vi "Main.vi"(11 "Module Admin":refnum<class "Delacor_lib_QMH_Module Admin.lvclass">) -> ()   [LabVIEW 2023, in "RT Main.lvlib"]
doc: "This template is based off of the Queued Message Handler design pattern and the Queued Message Handler project template that ships with LabVIEW.\n\nThe main difference is that the queue is private to this module and communication between modules is performed via Broadcast and Request events.\n\nRequest events are wrapped in public API methods and are handled in the Event Handling Loop (EHL) of this VI. Any module can register for Broadcast events sent by this module. The EHL generates messages based on user interface actions.\n\nThe Message Handling Loop (MHL) processes messages generated by the EHL, or by other messages. The messages are string values, so new messages can be added easily to the Message Cases case structure in the MHL. Each message cluster can also provide an optional value for Message Data, which is a variant that can be converted to whatever message-specific data is required.\n_____\nBased on DQMH Dev Tools: Project Template 7.1.2.1547."
uses:
  RT Main.lvlib
  <vilib>/Delacor/Delacor QMH/Libraries/Module Admin_class/Delacor_lib_QMH_Module Admin.lvclass
  Module Data--cluster.ctl
  <vilib>/myRIO/Instrument Drivers/Onboard IO/AI/typedefs/AI Reference.ctl
  <vilib>/myRIO/Common/Instrument Driver Framework/Utilities/typedefs/myRIO Generic Hardware Reference.ctl
  <vilib>/myRIO/Common/Instrument Driver Framework/Utilities/typedefs/Hardware Version Enum.ctl
  <vilib>/myRIO/Common/Instrument Driver Framework/Utilities/typedefs/myRIO v1.0 Reference.ctl
  <vilib>/myRIO/Common/Instrument Driver Framework/Utilities/typedefs/Generic FPGA Reference.ctl
  <vilib>/myRIO/Common/Instrument Driver Framework/myRIO v1.0/AI/typedefs/AI Channels List.ctl
  <vilib>/myRIO/Common/Instrument Driver Framework/myRIO v1.0/AI/typedefs/AI Channels Enum.ctl
  <vilib>/myRIO/Common/Instrument Driver Framework/Utilities/typedefs/Analog Scaling Constants List.ctl
  <vilib>/myRIO/Common/Instrument Driver Framework/Utilities/typedefs/Analog Scaling Constants.ctl
  <vilib>/myRIO/Instrument Drivers/Onboard IO/DIO/typedefs/DIO Reference.ctl
  <vilib>/myRIO/Common/Instrument Driver Framework/myRIO v1.0/DIO/typedefs/DIO Channels List.ctl
  <vilib>/myRIO/Common/Instrument Driver Framework/myRIO v1.0/DIO/typedefs/DIO Channels Enum.ctl
  Modules Launched.ctl
  Hardware Monitoring.ctl
  Stop Argument--cluster.ctl
  <vilib>/Delacor/Delacor QMH/Libraries/Message Queue_class/Delacor_lib_QMH_Message Queue.lvclass/Delacor_lib_QMH_Message Queue.ctl
  <vilib>/Delacor/Delacor QMH/Libraries/Module Admin_class/Delacor_lib_QMH_Module Admin.lvclass/Delacor_lib_QMH_Module Admin.ctl
  Control Loop Cluster.ctl
  Data Cluster.ctl
  <vilib>/Delacor/Delacor QMH/Libraries/Message Queue_class/Delacor_lib_QMH_Enqueue Message (Single).vi
  <vilib>/Delacor/Delacor QMH/Libraries/Module Admin_class/Delacor_lib_QMH_Get External Launch.vi
  <vilib>/nisyscfg/Close (System).vi
  Control Loop.vi
  <vilib>/Delacor/Delacor QMH/Libraries/Message Queue_class/Delacor_lib_QMH_Message Queue.lvclass
  Analog Input/Analog Input.lvlib
  <vilib>/myRIO/Instrument Drivers/Onboard IO/AI/AI.lvlib
  <vilib>/nisyscfg/nisyscfg.lvlib
  <resource>/objmgr/nicriosae.rc
  <resource>/objmgr/nisysapi.rc
  Digital Inputs/Digital Inputs.lvlib
  <vilib>/myRIO/Instrument Drivers/Onboard IO/DIO/DIO.lvlib
  Modules/TDMS/TDMS.lvlib
  UDP RT/UDP RT.lvlib
panel:
  out "error out":errorcluster
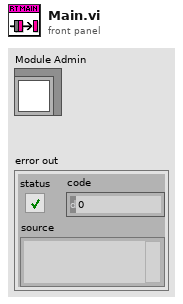
[diagram p1: front panel]
types:
  T1 = typedef "RT Main.lvlib/Request Events--cluster.ctl" = cluster{"Stop Module":refnum<user-event>, "Show Panel":refnum<user-event>, "Hide Panel":refnum<user-event>, "Get Module Execution Status":refnum<user-event>, "Show Diagram":refnum<user-event>, "Private.Launch Control Loop":refnum<user-event>, "Private.RT FIFO Ref":refnum<user-event>}
  T2 = typedef "Analog Input.lvlib/Broadcast Events--cluster.ctl" = cluster{"Module Did Init":refnum<user-event>, "Status Updated":refnum<user-event>, "Error Reported":refnum<user-event>, "Module Did Stop":refnum<user-event>, "Update Module Execution Status":refnum<user-event>, "AI Input Reference":refnum<user-event>}
  T3 = typedef "Digital Inputs.lvlib/Broadcast Events--cluster.ctl" = cluster{"Module Did Init":refnum<user-event>, "Status Updated":refnum<user-event>, "Error Reported":refnum<user-event>, "Module Did Stop":refnum<user-event>, "Update Module Execution Status":refnum<user-event>, "Send DI Reference":refnum<user-event>}
  T4 = typedef "TDMS.lvlib/Broadcast Events--cluster.ctl" = cluster{"Module Did Init":refnum<user-event>, "Status Updated":refnum<user-event>, "Error Reported":refnum<user-event>, "Module Did Stop":refnum<user-event>, "Update Module Execution Status":refnum<user-event>}
  T5 = typedef "UDP RT.lvlib/Broadcast Events--cluster.ctl" = cluster{"Module Did Init":refnum<user-event>, "Status Updated":refnum<user-event>, "Error Reported":refnum<user-event>, "Module Did Stop":refnum<user-event>, "Update Module Execution Status":refnum<user-event>, "Send UDP Info to TL":refnum<user-event>}
  T6 = typedef "RT Main.lvlib/Module Data--cluster.ctl" = cluster{"Status":string, "Current Directory":path, "AI Reference":T7, "DIO Reference":T16, "UDP Info":cluster{"IP Host":string, "Port RT":u16, "Port Host":u16, "connection ID":refnum<k16>}, "Modules Launched":T19, "RTFIFO HW":refnum<k33>}
  T7 = typedef "AI.lvlib/AI Reference.ctl" = cluster{"myRIO Reference":T8, "AI Channels List":T12, "AI Scaling Constants List":T14}
  T8 = typedef "myRIO Generic Hardware Reference.ctl" = cluster{"myRIO Model":T9, "myRIO Hardware Reference":T10}
  T9 = typedef "Hardware Version Enum.ctl" = enum16{"Unknown", "myRIO-1900", "myRIO-1950", "roboRIO", "NI ELVIS RIO CM", "ELVIS III"}
  T10 = typedef "myRIO v1.0 Reference.ctl" = cluster{"Generic FPGA Reference":T11, "Allow multiple opens":bool}
  T11 = typedef "Generic FPGA Reference.ctl" = refnum<k20>
  T12 = typedef "AI Channels List.ctl" = T13[]
  T13 = typedef "AI Channels Enum.ctl" = enum16{"Not Connected", "AudioIn/Left", "AudioIn/Right", "C/AI0", "C/AI1", "A/AI0", "A/AI1", "A/AI2", "A/AI3", "A/AI4", "A/AI5", "A/AI6", "A/AI7", "B/AI0", "B/AI1", "B/AI2", "B/AI3", "B/AI4", "B/AI5", "B/AI6", "B/AI7", "AI/AI0", "AI/AI1", "AI/AI2", "AI/AI3", "A/AI0 (DIFF)", "A/AI1 (DIFF)", "A/AI2 (DIFF)", "A/AI3 (DIFF)", "B/AI0 (DIFF)", "B/AI1 (DIFF)", "B/AI2 (DIFF)", "B/AI3 (DIFF)"}
  T14 = typedef "Analog Scaling Constants List.ctl" = T15[]
  T15 = typedef "Analog Scaling Constants.ctl" = cluster{"LSB Weight (Volts)":dbl, "Offset (Volts)":dbl, "Signed?":bool}
  T16 = typedef "DIO.lvlib/DIO Reference.ctl" = cluster{"myRIO Reference":T8, "DIO Channels List":T17}
  T17 = typedef "DIO Channels List.ctl" = T18[]
  T18 = typedef "DIO Channels Enum.ctl" = enum16{"Not Connected", "C/DIO0", "C/DIO1", "C/DIO2", "C/DIO3", "C/DIO4", "C/DIO5", "C/DIO6", "C/DIO7", "A/DIO0", "A/DIO1", "A/DIO2", "A/DIO3", "A/DIO4", "A/DIO5", "A/DIO6", "A/DIO7", "A/DIO8", "A/DIO9", "A/DIO10", "A/DIO11", "A/DIO12", "A/DIO13", "A/DIO14", "A/DIO15", "A/DIO16", "A/DIO17", "A/DIO18", "A/DIO19", "B/DIO0", "B/DIO1", "B/DIO2", "B/DIO3", "B/DIO4", "B/DIO5", "B/DIO6", "B/DIO7", "B/DIO8", "B/DIO9", "B/DIO10", "B/DIO11", "B/DIO12", "B/DIO13", "B/DIO14", "B/DIO15", "B/DIO16", "B/DIO17", "B/DIO18", "B/DIO19", "LED0", "LED1", "LED2", "LED3", "Button0", "DIO/DIO0", "DIO/DIO1", "DIO/DIO2", "DIO/DIO3", "DIO/DIO4", "DIO/DIO5", "DIO/DIO6", "DIO/DIO7", "DIO/DIO8", "DIO/DIO9", "SPI/CS0", "SPI/CS1", "SPI/CS2", "SPI/CS3", "LED RADIO (Green)", "LED RADIO (Red)", "LED COMM (Green)", "LED COMM (Red)", "LED MODE (Green)", "LED MODE (Red)"}
  T19 = typedef "RT Main.lvlib/Modules Launched.ctl" = cluster{"AI Input":bool, "DI Input":bool, "TDMS Module":bool, "UDP Module":bool}
  T20 = typedef "RT Main.lvlib/Hardware Monitoring.ctl" = cluster{"Memory RAM Free (%)":dbl, "Memory ROM Free (%)":dbl, "CPU 1 (%)":u32, "CPU 2 (%)":u32}
  T21 = enum32{"invalid lock state", "Not Locked", "Locked (No Password)", "Password-protected"}
  T22 = typedef "RT Main.lvlib/Stop Argument--cluster.ctl" = cluster{"Origin":string, "Exit via Stop Module Req?":bool, "Wait for Module to stop?":bool}
  T23 = cluster{"IP Host":string, "Port RT":u16, "Port Host":u16, "connection ID":refnum<k16>}
  T24 = typedef "RT Main.lvlib/Control Loop Cluster.ctl" = cluster{"AI Reference":T7, "DIO Reference":T16, "Data Cluster":T25, "TDMS Record?":bool, "Writing?":bool, "UDP Info":cluster{"IP Host":string, "Port RT":u16, "Port Host":u16, "connection ID":refnum<k16>}, "RT FIFO HW":refnum<k33>}
  T25 = typedef "RT Main.lvlib/Data Cluster.ctl" = cluster{"Analog Input":dbl[], "Digital Inputs":bool[], "U32":u32[]}
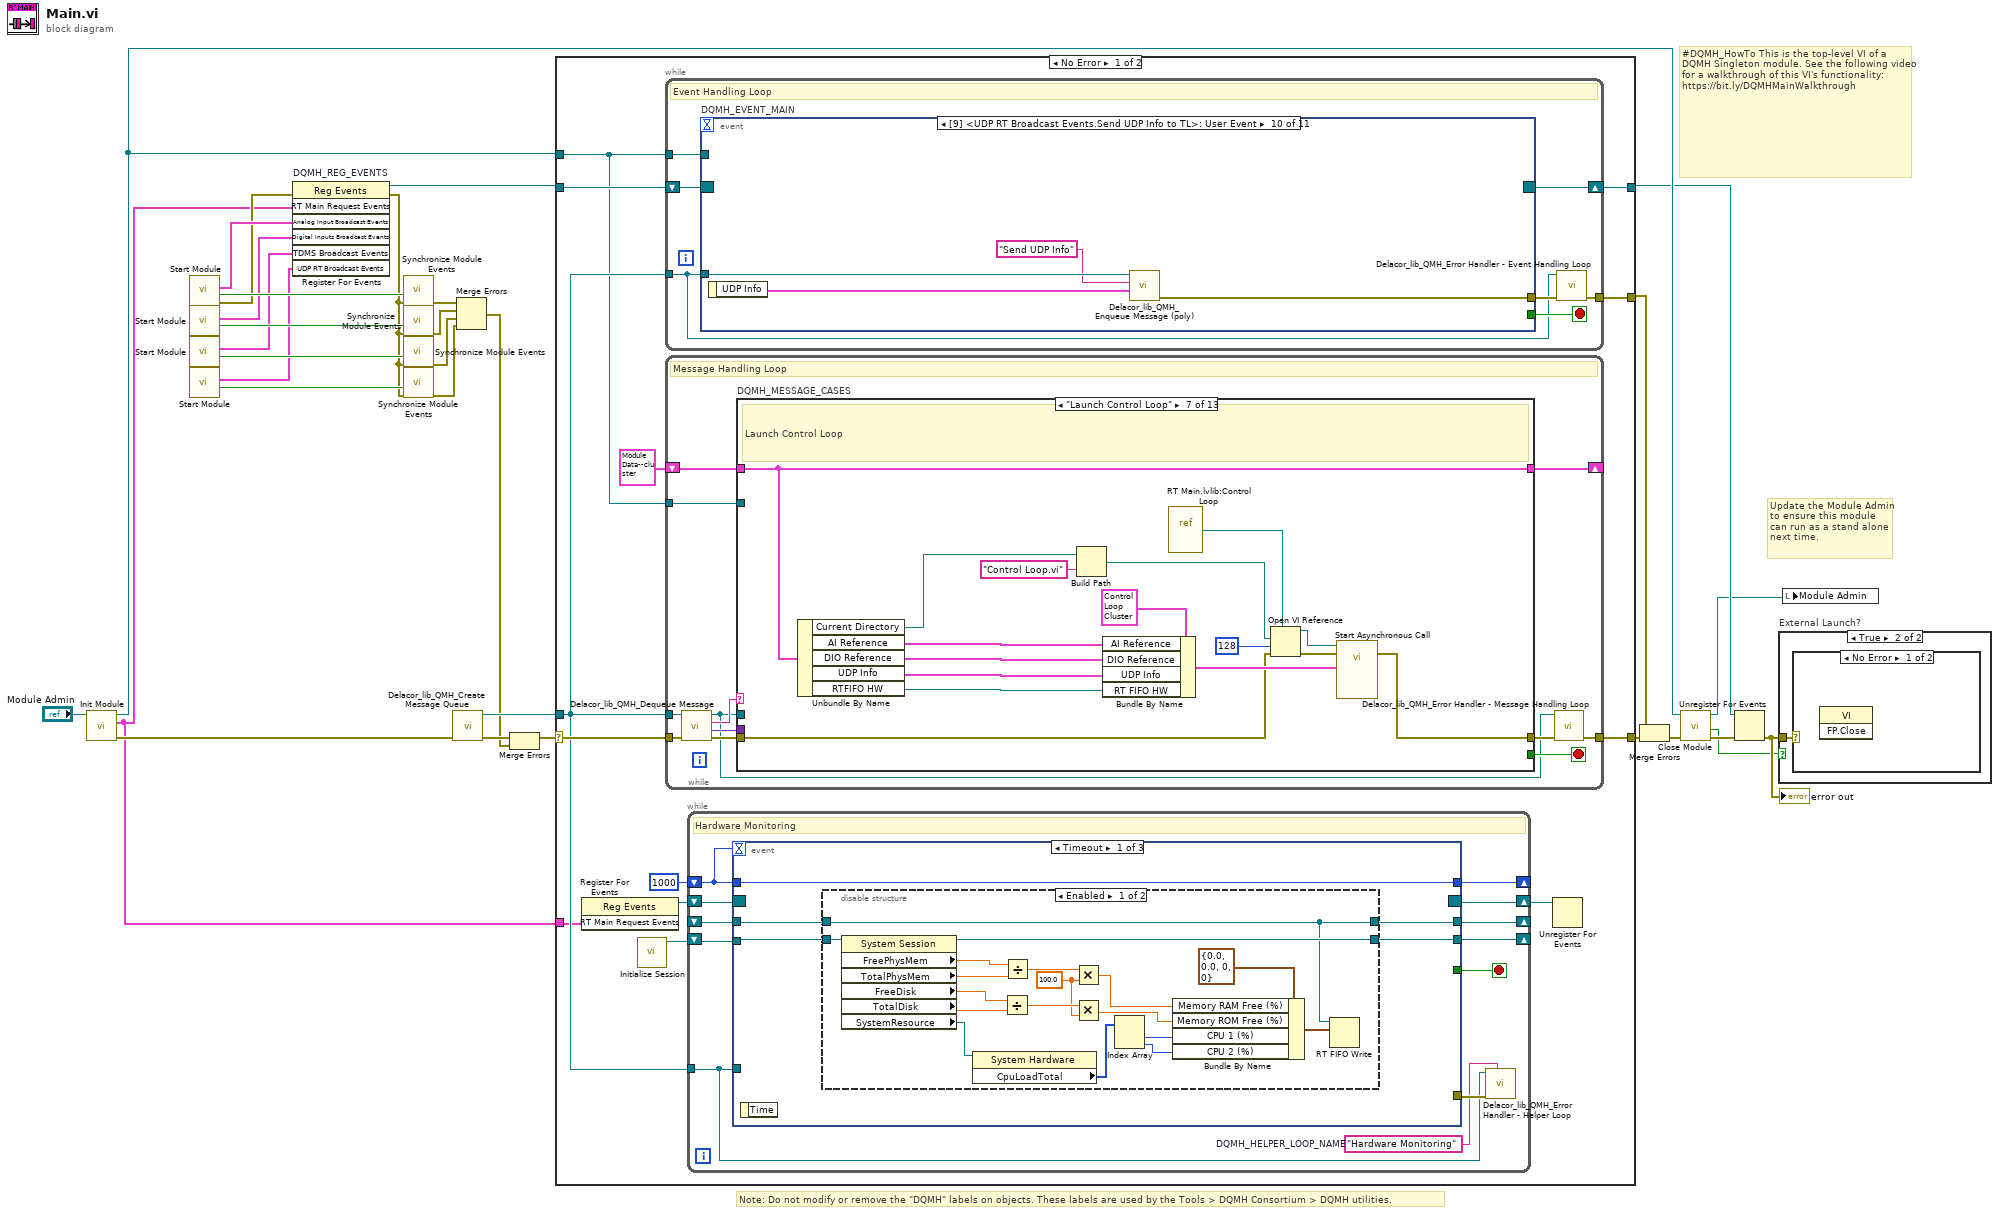
[diagram p0: block diagram]
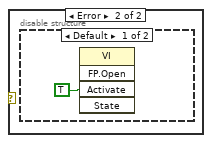
[diagram p3: hidden frame]
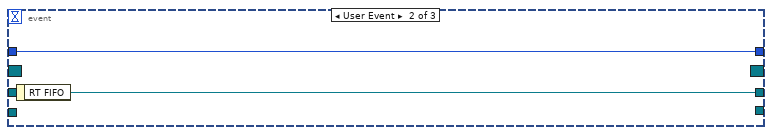
[diagram p6: hidden frame]
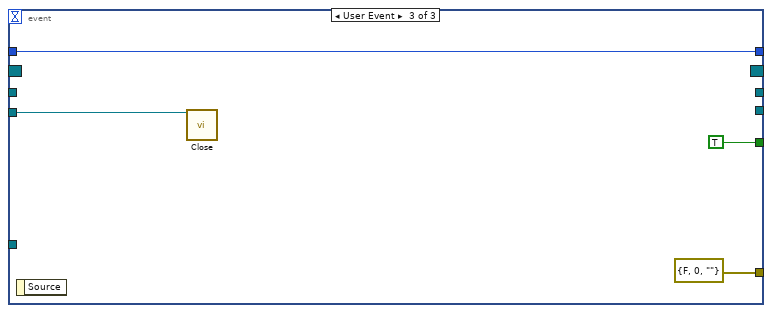
[diagram p7: hidden frame]
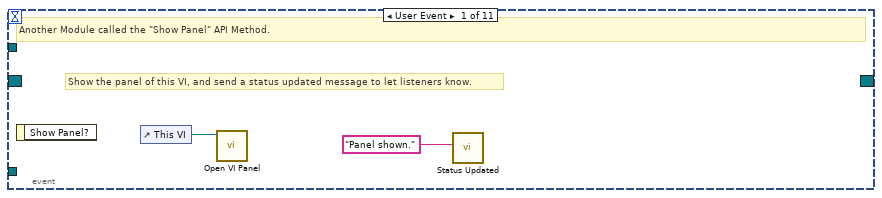
[diagram p8: hidden frame]
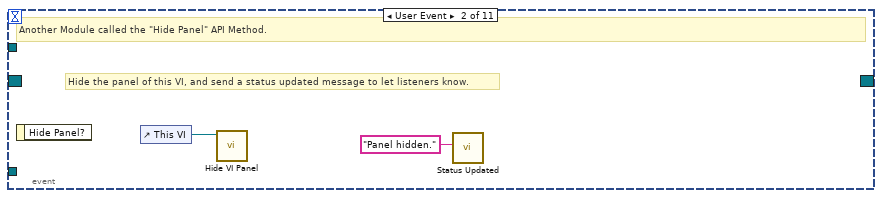
[diagram p9: hidden frame]
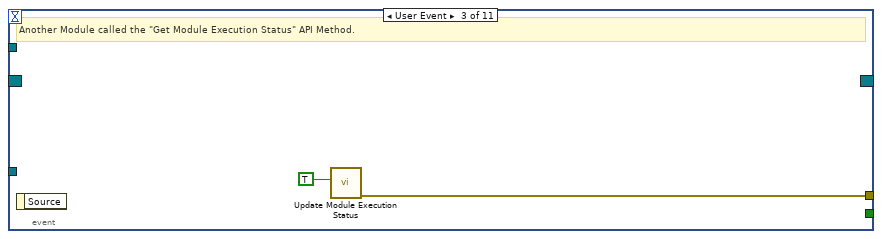
[diagram p10: hidden frame]
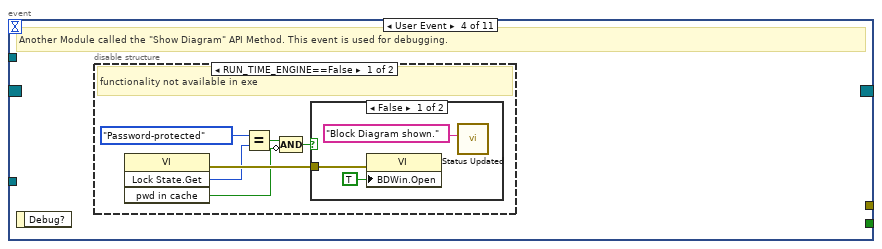
[diagram p11: hidden frame]
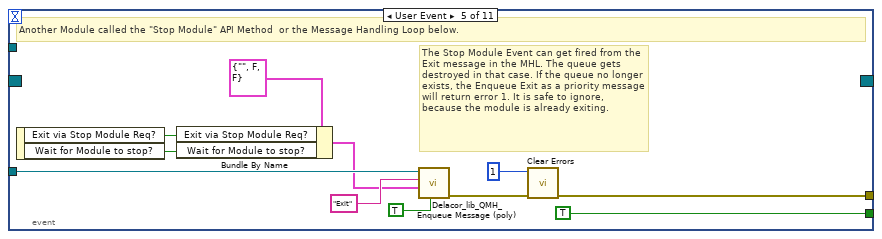
[diagram p14: hidden frame]
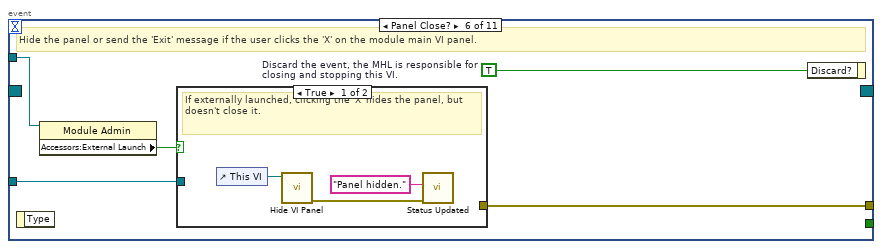
[diagram p15: hidden frame]
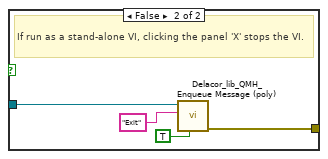
[diagram p16: hidden frame]
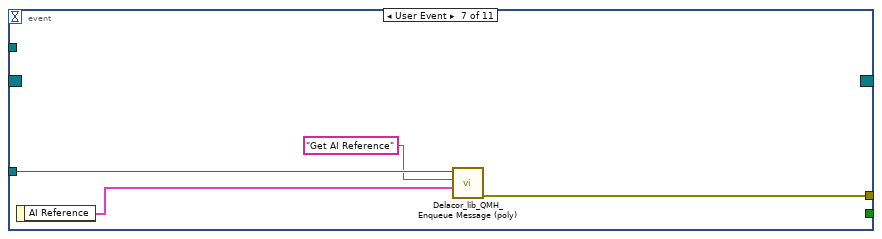
[diagram p17: hidden frame]
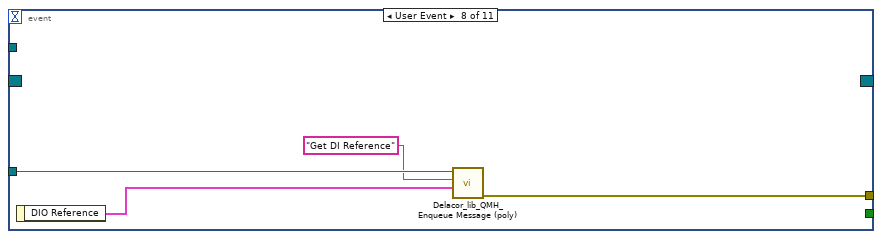
[diagram p18: hidden frame]
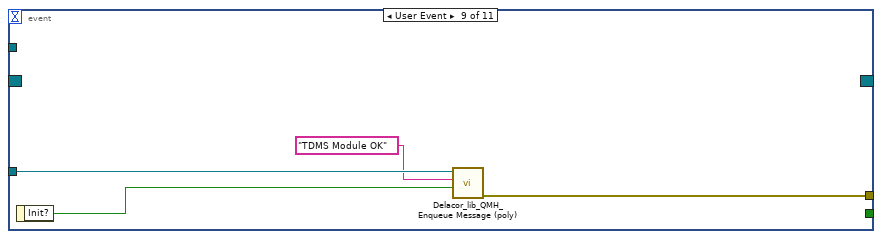
[diagram p19: hidden frame]
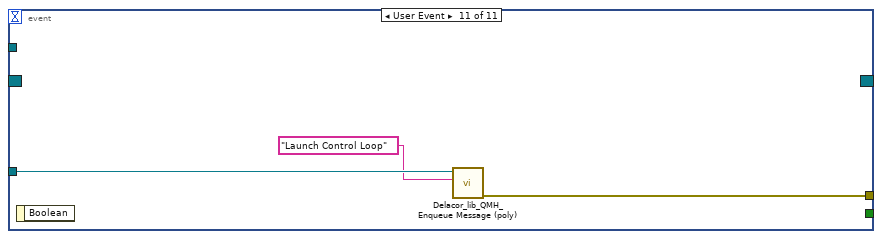
[diagram p20: hidden frame]
diagram:
  # "#DQMH_HowTo This is the top-level VI of a DQMH Singleton module. See the following video for a walkthrough of this VI's functionality: https://bit.ly/DQMHMainWalkthrough"
  # "Note: Do not modify or remove the \"DQMH\" labels on objects. These labels are used by the Tools > DQMH Consortium > DQMH utilities."
  # "Update the Module Admin to ensure this module can run as a stand alone next time."
  n1 = call "Init Module.vi"("Singleton Module Admin in"="Module Admin") -> ("error out"=w30:errorcluster, "RT Main Request Events"=w11:T1, "Singleton Module Admin out"=w23:refnum<class "Delacor_lib_QMH_Module Admin.lvclass">)  [unwired: 8 in]
  n2 = call "Start Module.vi"() -> ("error out"=w14:errorcluster, "Wait for Event Sync?"=w15:bool, "Analog Input Broadcast Events"=w16:T2)  [unwired: 7 in, 2 out]
  n3 = call "Start Module.vi"() -> ("Wait for Event Sync?"=w10:bool, "Digital Inputs Broadcast Events"=w9:T3)  [unwired: 7 in, 3 out]
  n4 = call "Start Module.vi"() -> ("Wait for Event Sync?"=w6:bool, "TDMS Broadcast Events"=w7:T4)  [unwired: 8 in, 2 out]
  n5 = call "Start Module.vi"() -> ("Wait for Event Sync?"=w4:bool, "UDP RT Broadcast Events"=w3:T5)  [unwired: 7 in, 3 out]
  n6 = register-events "DQMH_REG_EVENTS"(error in=w14, w11, w16, w9, w7, w3) -> (reference out=w21:refnum<event-registration>, error out=w2:errorcluster)  [unwired: 1 in]
  n7 = call "Synchronize Module Events.vi"("error in"=w2, "Wait for Event Sync?"=w15) -> ("error out"=w13:errorcluster)  [unwired: 9 in]
  n8 = call "Synchronize Module Events.vi"("error in"=w2, "Wait for Event Sync?"=w10) -> ("error out"=w8:errorcluster)  [unwired: 9 in]
  n9 = call "Synchronize Module Events.vi"("error in"=w2, "Wait for Event Sync?"=w6) -> ("error out"=w5:errorcluster)  [unwired: 9 in]
  n10 = call "Synchronize Module Events.vi"("error in"=w2, "Wait for Event Sync?"=w4) -> ("error out"=w1:errorcluster)  [unwired: 9 in]
  n11 = call <vilib>:"Delacor_lib_QMH_Create Message Queue.vi"("error in"=w30) -> ("error out"=w25:errorcluster, "Message Queue"=w20:refnum<class "Delacor_lib_QMH_Message Queue.lvclass">)  [unwired: 9 in]
  n12 = Merge Errors(w13, w8, w5, w1) -> (w12:errorcluster)
  n13 = Merge Errors(w25, w12) -> (w24:errorcluster)
  n14 = case shown="No Error" w24 {
    selector: w24 -> [w42 w314]
    tunnel: [w44 w313] -> w31
    tunnel: [w41 w312] -> w22
    tunnel: w21 -> [w39 w312]
    tunnel: w20 -> [w38 w307]
    tunnel: [w43 _] -> w28
    tunnel: w23 -> [w37 w308]
    tunnel: w11 -> [w36 _]
    frame No Error {
      n15 = register-events ("DQMH_HELPER_REGFOREVENTS")(w36) -> (reference out=w34:refnum<event-registration>)  [unwired: 2 in, 1 out]
      n16 = call <vilib>:"Initialize Session.vi"() -> ("Session out"=w32:refnum<k21>)  [unwired: 10 in, 1 out]
      n17 = while {
        tunnel: w38 -> [w87]
        shift-right: [w90] -> w41
        shift-left: w39 -> [w91]
        tunnel: [w92] -> w43
        tunnel: w37 -> [w88]
        stop <- w89 stop-if-true
        # "Event Handling Loop"
        n18 = event "DQMH_EVENT_MAIN" shown="[9] <UDP RT Broadcast Events.Send UDP Info to TL>: User Event" {
          selector: w91 -> [_ _ _ _ _ _ _ _ _ _ _]
          dyn-events: [_ _ _ _ _ _ _ _ _ _ _] -> w90
          timeout: _ -> [_ _ _ _ _ _ _ _ _ _ _]
          tunnel: [_ _ _ _ TRUE ("Discard?") _ _ _ _ _ _] -> w89
          tunnel: w87 -> [_ _ _ _ w115 w122 w135 w139 w143 w147 w150]
          tunnel: [_ _ w99 _ w118 w124 w132 w136 w140 w144 w148] -> w93
          tunnel: w88 -> [_ _ _ _ _ w121 _ _ _ _ _]
          event User Event {
            # "Show the panel of this VI, and send a status updated message to let listeners know."
            # "Another Module called the \"Show Panel\" API Method."
            n19 = event-data() -> ()  [unwired: 1 in, 1 out]
            n20 = control-ref of="This VI"() -> (w95:refnum<vi>)
            n21 = call "Open VI Panel.vi"("VI"=w95) -> ()  [unwired: 10 in, 1 out]
            n22 = call "Status Updated.vi"("Status"="Panel shown." ("format string")) -> ()  [unwired: 10 in, 1 out]
          }
          event User Event {
            # "Hide the panel of this VI, and send a status updated message to let listeners know."
            # "Another Module called the \"Hide Panel\" API Method."
            n23 = event-data() -> ()  [unwired: 1 in, 1 out]
            n24 = control-ref of="This VI"() -> (w97:refnum<vi>)
            n25 = call "Hide VI Panel.vi"("VI"=w97) -> ()  [unwired: 10 in, 1 out]
            n26 = call "Status Updated.vi"("Status"="Panel hidden." ("format string")) -> ()  [unwired: 10 in, 1 out]
          }
          event User Event {
            # "Another Module called the \"Get Module Execution Status\" API Method."
            n27 = event-data() -> ()  [unwired: 1 in, 1 out]
            n28 = call "Update Module Execution Status.vi"("Running?"=TRUE) -> ("error out"=w99:errorcluster)  [unwired: 10 in]
          }
          event User Event {
            # "Another Module called the \"Show Diagram\" API Method. This event is used for debugging."
            n29 = event-data() -> ()  [unwired: 1 in, 1 out]
            n30 = disable-structure shown="RUN_TIME_ENGINE==False" {
              frame condition #0 (active) {
                # "functionality not available in exe"
                n31 = invoke on="Invoke Node" class="VI" method="Lock State.Get"() -> (error out=w105:errorcluster, "Get Lock State"=w104:T21, "pwd in cache"=w101:bool)  [unwired: 4 in, 1 out]
                n32 = Equal?(x=T21."Password-protected", y=w104) -> (x = y?=w102:bool)
                n33 = Compound Arithmetic op=AND(w102, invert w101) -> (w100:bool)
                n34 = case shown="False" w100 {
                  tunnel: w105 -> [w108 _]
                  frame False {
                    n35 = property on="Property Node" class="VI"(error in=w108, "BDWin.Open"=TRUE ("Block Diagram Window:Open")) -> ()  [unwired: 1 in, 2 out]
                    n36 = call "Status Updated.vi"("Status"="Block Diagram shown." ("format string")) -> ()  [unwired: 10 in, 1 out]
                  }
                  frame True {
                    # "Password-protected VI, and the password is not in the cache. Do not show the diagram."
                  }
                }
              }
              frame condition #1 {
              }
            }
          }
          event User Event {
            # "The Stop Module Event can get fired from the Exit message in the MHL. The queue gets destroyed in that case. If the queue no longer exists, the Enqueue Exit as a priority message will return error 1. It is safe to ignore, because the module is already exiting."
            # "Another Module called the \"Stop Module\" API Method  or the Message Handling Loop below."
            n37 = event-data() -> ("Exit via Stop Module Req?"=w111:bool, "Wait for Module to stop?"=w110:bool)  [unwired: 1 in]
            n38 = Bundle By Name(cluster=T22 {"Origin"="", "Exit via Stop Module Req?"=FALSE, "Wait for Module to stop?"=FALSE} ("Stop Argument"), "Exit via Stop Module Req?"=w111, "Wait for Module to stop?"=w110) -> (w109:T22)
            n39 = call-poly <vilib>:"Delacor_lib_QMH_Enqueue Message (poly).vi"("Priority Message? (F)"=TRUE, "Message Data"=w109, "Message"="Exit", "Message Queue in"=w115) -> ("error out"=w119:errorcluster)  [unwired: 6 in, 1 out]
            n40 = call <vilib>:"Clear Errors.vi"("error in (no error)"=w119, "specific error code to clear (0: all)"=1) -> ("error out"=w118:errorcluster)  [unwired: 4 in, 1 out]
          }
          event Panel Close? {
            w123 = TRUE  # Discard the event, the MHL is responsible for closing and stopping this VI.
            # "Hide the panel or send the 'Exit' message if the user clicks the 'X' on the module main VI panel."
            n41 = event-data() -> ()  [unwired: 1 in, 1 out]
            n42 = property on="Property Node" class="Module Admin"(reference=w121) -> ("Accessors:External Launch"=w120:bool)  [unwired: 1 in, 2 out]
            n43 = case shown="True" w120 {
              tunnel: w122 -> [_ w130]
              tunnel: [_ w131] -> w124
              frame True {
                # "If externally launched, clicking the 'X' hides the panel, but doesn't close it."
                n44 = control-ref of="This VI"() -> (w127:refnum<vi>)
                n45 = call "Hide VI Panel.vi"("VI"=w127) -> ("error out"=w125:errorcluster)  [unwired: 10 in]
                n46 = call "Status Updated.vi"("error in"=w125, "Status"="Panel hidden." ("format string")) -> ()  [unwired: 9 in, 1 out]
              }
              frame False {
                # "If run as a stand-alone VI, clicking the panel 'X' stops the VI."
                n47 = call-poly <vilib>:"Delacor_lib_QMH_Enqueue Message (poly).vi"("Priority Message? (F)"=TRUE, "Message"="Exit", "Message Queue in"=w130) -> ("error out"=w131:errorcluster)  [unwired: 7 in, 1 out]
              }
            }
            n48 = event-data ("Event Filter Node")("Discard?"=w123) -> ()  [unwired: 1 in, 1 out]
          }
          event User Event {
            n49 = event-data() -> ("AI Reference"=w133:T7)  [unwired: 1 in]
            n50 = call-poly <vilib>:"Delacor_lib_QMH_Enqueue Message (poly).vi"("Message Data"=w133, "Message"="Get AI Reference", "Message Queue in"=w135) -> ("error out"=w132:errorcluster)  [unwired: 7 in, 1 out]
          }
          event User Event {
            n51 = event-data() -> ("DIO Reference"=w137:T16)  [unwired: 1 in]
            n52 = call-poly <vilib>:"Delacor_lib_QMH_Enqueue Message (poly).vi"("Message Data"=w137, "Message"="Get DI Reference", "Message Queue in"=w139) -> ("error out"=w136:errorcluster)  [unwired: 7 in, 1 out]
          }
          event User Event {
            n53 = event-data() -> ("Init?"=w141:bool)  [unwired: 1 in]
            n54 = call-poly <vilib>:"Delacor_lib_QMH_Enqueue Message (poly).vi"("Message Data"=w141, "Message"="TDMS Module OK", "Message Queue in"=w143) -> ("error out"=w140:errorcluster)  [unwired: 7 in, 1 out]
          }
          event User Event {
            n55 = event-data() -> ("UDP Info"=w145:T23)  [unwired: 1 in]
            n56 = call-poly <vilib>:"Delacor_lib_QMH_Enqueue Message (poly).vi"("Message Data"=w145, "Message"="Send UDP Info", "Message Queue in"=w147) -> ("error out"=w144:errorcluster)  [unwired: 7 in, 1 out]
          }
          event User Event {
            n57 = event-data() -> ()  [unwired: 1 in, 1 out]
            n58 = call-poly <vilib>:"Delacor_lib_QMH_Enqueue Message (poly).vi"("Message"="Launch Control Loop", "Message Queue in"=w150) -> ("error out"=w148:errorcluster)  [unwired: 8 in, 1 out]
          }
        }
        n59 = call-dynamic "Delacor_lib_QMH_Error Handler - Event Handling Loop.vi"("error in"=w93, "Message Queue in"=w87) -> ("dup error in"=w92:errorcluster)  [unwired: 8 in, 1 out]
      }
      n60 = while {
        tunnel: w38 -> [w151]
        shift-right: [w159] -> _
        shift-left: T6 {"Status"="", "Current Directory"=path "", "AI Reference"={"myRIO Reference"={"myRIO Model"=enum."Unknown", "myRIO Hardware Reference"={"Generic FPGA Reference"=refnum, "Allow multiple opens"=FALSE}}, "AI Channels List"=[], "AI Scaling Constants List"=[]}, "DIO Reference"={"myRIO Reference"={"myRIO Model"=enum."Unknown", "myRIO Hardware Reference"={"Generic FPGA Reference"=refnum, "Allow multiple opens"=FALSE}}, "DIO Channels List"=[]}, "UDP Info"={"IP Host"="", "Port RT"=0, "Port Host"=0, "connection ID"=refnum}, "Modules Launched"={"AI Input"=FALSE, "DI Input"=FALSE, "TDMS Module"=FALSE, "UDP Module"=FALSE}, "RTFIFO HW"=refnum} ("Data Cluster") -> [w160]
        tunnel: w42 -> [w162]
        tunnel: [w154] -> w44
        tunnel: w37 -> [w155]
        stop <- w158 stop-if-true
        # "Message Handling Loop"
        n61 = call-dynamic "Delacor_lib_QMH_Dequeue Message.vi"("error in"=w162, "Message Queue in"=w151) -> ("error out"=w161:errorcluster, "Message Data"=w156:variant, "Message"=w157:string, "Message Queue out"=w152:refnum<class "Delacor_lib_QMH_Message Queue.lvclass">)  [unwired: 6 in]
        n62 = case "DQMH_MESSAGE_CASES" shown="\"Launch Control Loop\"" w157 {
          selector: w157 -> [_ _ _ _ _ _ _ _ _ _ _ _ w302]
          tunnel: w152 -> [_ _ _ _ _ _ _ _ _ _ w268 w291 _]
          tunnel: w161 -> [w176 w178 w190 w205 w220 w231 w243 w253 w255 w264 w275 w296 w305]
          tunnel: [w163 w178 w179 w196 w211 w224 w244 w252 w255 w263 w271 w282 w306] -> w153
          tunnel: w160 -> [w168 w177 w185 w202 w217 w229 w250 w251 w254 w261 w270 w290 w303]
          tunnel: [w169 w177 w184 w201 w216 w228 w250 w251 w254 w261 w270 w290 w303] -> w159
          tunnel: [_ _ _ _ _ _ _ _ _ _ _ w289 _] -> w158
          tunnel: w156 -> [_ _ w189 w204 w219 _ _ _ _ _ w269 w288 _]
          tunnel: w155 -> [w174 _ _ _ _ _ _ _ _ _ w267 w283 _]
          frame "Initialize" {
            # "Initialize - Any operation that needs to be done before the module can receive messages. Synchronize Caller Events.vi will inform Start Module.vi that the module has launched and is ready to receive messages. Module Did Init.vi will broadcast that the module initialized."
            n63 = call "Synchronize Caller Events.vi"("error in"=w176, "Singleton Module Admin in"=w174) -> ("error out"=w175:errorcluster)  [unwired: 8 in, 1 out]
            n64 = call "Module Name--constant.vi"() -> ("Module Name"=w172:string)  [unwired: 11 in]
            n65 = call "Module Did Init.vi"("error in"=w175, "Initialized?"=TRUE, "Origin"=w172) -> ("error out"=w166:errorcluster)  [unwired: 8 in]
            n66 = Current VI's Path() -> (path=w171:path)
            n67 = Strip Path(path=w171) -> (stripped path=w170:path)  [unwired: 1 out]
            n68 = RT FIFO Create(1:T20 {"Memory RAM Free (%)"=0.0, "Memory ROM Free (%)"=0.0, "CPU 1 (%)"=0, "CPU 2 (%)"=0} ("Hardware Monitoring"), 3:w166) -> (8:w165:refnum<k33>, 11:w164:errorcluster)  [unwired: 6 in, 1 out]
            n69 = Bundle By Name(cluster=w168, "Current Directory"=w170, "RTFIFO HW"=w165) -> (w169:T6)
            n70 = call "Get RT FIFO HW Ref.vi"("error in"=w164, "RT FIFO"=w165) -> ("error out"=w163:errorcluster)  [unwired: 9 in]
          }
          frame "---Module Specific---" {
            # "Separator -- The following cases handle messages specific to this Module."
          }
          frame "Get AI Reference" {
            # "Get AI Reference"
            n71 = Variant To Data(error in=w190, type=T7 {"myRIO Reference"={"myRIO Model"=enum."Unknown", "myRIO Hardware Reference"={"Generic FPGA Reference"=refnum, "Allow multiple opens"=FALSE}}, "AI Channels List"=[], "AI Scaling Constants List"=[]} ("AI Reference"), Variant=w189) -> (data=w187:T7, error out=w180:errorcluster)
            n72 = Bundle By Name(cluster=w185, "Modules Launched.AI Input"=TRUE, "AI Reference"=w187) -> (w184:T6)
            n73 = Unbundle By Name(w184) -> ("Modules Launched"=w183:T19)
            n74 = Cluster To Array(cluster=w183) -> (array=w182:bool[])
            n75 = And Array Elements(Boolean array=w182) -> (logical AND=w181:bool)
            n76 = case shown="True" w181 {
              tunnel: w180 -> [w191 w192]
              tunnel: [w191 w193] -> w179
              frame False {
              }
              frame True {
                n77 = call "Launch Control Loop.vi"("error in"=w192) -> ("error out"=w193:errorcluster)  [unwired: 10 in]
              }
            }
          }
          frame "Get DI Reference" {
            # "Get DI Reference"
            n78 = Variant To Data(error in=w205, type=T16 {"myRIO Reference"={"myRIO Model"=enum."Unknown", "myRIO Hardware Reference"={"Generic FPGA Reference"=refnum, "Allow multiple opens"=FALSE}}, "DIO Channels List"=[]} ("DIO Ref Out"), Variant=w204) -> (data=w194:T16, error out=w197:errorcluster)
            n79 = Bundle By Name(cluster=w202, "Modules Launched.DI Input"=TRUE ("Modules Launched.AI Input"), "DIO Reference"=w194) -> (w201:T6)
            n80 = Unbundle By Name(w201) -> ("Modules Launched"=w200:T19)
            n81 = Cluster To Array(cluster=w200) -> (array=w199:bool[])
            n82 = And Array Elements(Boolean array=w199) -> (logical AND=w198:bool)
            n83 = case shown="True" w198 {
              tunnel: w197 -> [w206 w207]
              tunnel: [w206 w208] -> w196
              frame False {
              }
              frame True {
                n84 = call "Launch Control Loop.vi"("error in"=w207) -> ("error out"=w208:errorcluster)  [unwired: 10 in]
              }
            }
          }
          frame "Send UDP Info" {
            # "Get DI Reference"
            n85 = Variant To Data(error in=w220, type=T23 {"IP Host"="", "Port RT"=0, "Port Host"=0, "connection ID"=refnum} ("Data Cluster"), Variant=w219) -> (data=w209:T23, error out=w212:errorcluster)
            n86 = Bundle By Name(cluster=w217, "Modules Launched.UDP Module"=TRUE ("Modules Launched.AI Input"), "UDP Info"=w209) -> (w216:T6)
            n87 = Unbundle By Name(w216) -> ("Modules Launched"=w215:T19)
            n88 = Cluster To Array(cluster=w215) -> (array=w214:bool[])
            n89 = And Array Elements(Boolean array=w214) -> (logical AND=w213:bool)
            n90 = case shown="True" w213 {
              tunnel: w212 -> [w221 w222]
              tunnel: [w221 w223] -> w211
              frame False {
              }
              frame True {
                n91 = call "Launch Control Loop.vi"("error in"=w222) -> ("error out"=w223:errorcluster)  [unwired: 10 in]
              }
            }
          }
          frame "TDMS Module OK" {
            # "TDMS Module OK"
            n92 = Bundle By Name(cluster=w229, "Modules Launched.TDMS Module"=TRUE ("Modules Launched.AI Input")) -> (w228:T6)
            n93 = Unbundle By Name(w228) -> ("Modules Launched"=w227:T19)
            n94 = Cluster To Array(cluster=w227) -> (array=w226:bool[])
            n95 = And Array Elements(Boolean array=w226) -> (logical AND=w225:bool)
            n96 = case shown="True" w225 {
              tunnel: w231 -> [w232 w233]
              tunnel: [w232 w234] -> w224
              frame False {
              }
              frame True {
                n97 = call "Launch Control Loop.vi"("error in"=w233) -> ("error out"=w234:errorcluster)  [unwired: 10 in]
              }
            }
          }
          frame "Launch Control Loop" {
            # "Launch Control Loop"
            n98 = Unbundle By Name(w250) -> ("Current Directory"=w241:path, "AI Reference"=w248:T7, "DIO Reference"=w237:T16, "UDP Info"=w236:T23, "RTFIFO HW"=w235:refnum<k33>)
            n99 = Build Path(base path=w241, name or relative path="Control Loop.vi") -> (appended path=w239:path)
            n100 = Bundle By Name(cluster=T24 {"AI Reference"={"myRIO Reference"={"myRIO Model"=enum."Unknown", "myRIO Hardware Reference"={"Generic FPGA Reference"=refnum, "Allow multiple opens"=FALSE}}, "AI Channels List"=[], "AI Scaling Constants List"=[]}, "DIO Reference"={"myRIO Reference"={"myRIO Model"=enum."Unknown", "myRIO Hardware Reference"={"Generic FPGA Reference"=refnum, "Allow multiple opens"=FALSE}}, "DIO Channels List"=[]}, "Data Cluster"={"Analog Input"=[], "Digital Inputs"=[], "U32"=[]}, "TDMS Record?"=FALSE, "Writing?"=FALSE, "UDP Info"={"IP Host"="", "Port RT"=0, "Port Host"=0, "connection ID"=refnum}, "RT FIFO HW"=refnum} ("Control Loop Cluster"), "AI Reference"=w248, "DIO Reference"=w237, "UDP Info"=w236, "RT FIFO HW"=w235) -> (w245:T24)
            n101 = vi-ref "RT Main.lvlib:Control Loop.vi"() -> (w247:refnum<vi>)
            n102 = Open VI Reference(type specifier VI Refnum (for type only)=w247, vi path=w239, options=128, error in (no error)=w243) -> (vi reference=w242:refnum<vi>, error out=w246:errorcluster)  [unwired: 2 in]
            n103 = call-by-ref "Start Asynchronous Call"(reference=w242, error in=w246, "Control Loop Cluster"=w245) -> (error out=w244:errorcluster)  [unwired: 10 in, 2 out]
          }
          frame "---Copy This Frame---" {
            # "Duplicate this frame when creating new messages.  Change this comment in the duplicated frame to describe this message."
            n104 = Merge Errors(w253) -> (w252:errorcluster)
          }
          frame "---Exit and Error Handling---" {
            # "Separator - The following cases handle errors and exit messages."
          }
          frame "Simulate MHL Error" {
            # "#DQMH_HowTo The 'Simulate MHL Error' button  illustrates how the MHL handles errors. This event is instructional in nature and can be removed."
            # "Simulate an error occurring at the MHL"
            n105 = call "Module Name--constant.vi"() -> ("Module Name"=w257:string)  [unwired: 11 in]
            n106 = Format Into String(format string="Simulated error originating at Message Handling Loop in %s", w257) -> (resulting string=w258:string)  [unwired: 2 in, 1 out]
            n107 = call <vilib>:"Error Cluster From Error Code.vi"("show call chain? (False)"=TRUE, "error message (\"\")"=w258, "error code (0)"=5001) -> ("error out"=w262:errorcluster)  [unwired: 6 in]
            n108 = Merge Errors(w264, w262) -> (w263:errorcluster)
          }
          frame "Error" {
            # "#DQMH_CodeRecommended - If the module is running in standalone mode (External Launch = FALSE), this code will pop up an error dialog and call the 'Exit' message if an error occurs. Add more fine-grained error management here."
            # "Error - Check the error message data and respond accordingly. This message is sent by the \"Error Handler\" VIs at the end of each loop in this application."
            n109 = property on="Property Node" class="Module Admin"(reference=w267) -> ("Accessors:External Launch"=w266:bool)  [unwired: 1 in, 2 out]
            n110 = Variant To Data(error in=w275, type=errorcluster {"status"=FALSE, "code"=0, "source"=""} ("error constant"), Variant=w269) -> (data=w265:errorcluster, error out=w273:errorcluster)
            n111 = local write "error out"(w265) -> ()
            n112 = call "Error Reported.vi"("Error"=w265) -> ()  [unwired: 10 in, 1 out]
            n113 = case shown="False" w266 {
              tunnel: [w280 _] -> w272
              tunnel: w268 -> [w278 _]
              tunnel: w265 -> [w279 _]
              frame False {
                n114 = disable-structure shown="Default" {
                  disable-tunnel: w279 -> [w281 _]
                  frame condition #0 (active) {
                    # "If the module is running standalone, then pop up an error dialog and call the \"Exit\" message."
                    n115 = call <vilib>:"Simple Error Handler.vi"("error in (no error)"=w281) -> ()  [unwired: 4 in, 5 out]
                  }
                  frame condition #1 {
                    # "To prevent the Simple Error Handler VI from being loaded (e.g. when deploying to a Real-Time target), add the Conditional Disable Symbol \"DQMH_Disable_SEH\" to your project and set it to TRUE."
                  }
                }
                n116 = call-poly <vilib>:"Delacor_lib_QMH_Enqueue Message (poly).vi"("Priority Message? (F)"=TRUE, "Message"="Exit", "Message Queue in"=w278) -> ("error out"=w280:errorcluster)  [unwired: 7 in, 1 out]
              }
              frame True {
                # "If the module was launched externally, calling the Error Reported broadcast VI is the only action performed by the \"Error\" message. The module's caller can then process the error appropriately."
              }
            }
            n117 = Merge Errors(w273, w272) -> (w271:errorcluster)
          }
          frame "Exit" {
            w287 = 91  # 91: not all Exit messages will have an argument
            w289 = TRUE  # Stop the VI
            # "Release the message queue reference"
            # "Exit - Exit the application."
            n118 = Variant To Data(error in=w296, type=T22 {"Origin"="", "Exit via Stop Module Req?"=FALSE, "Wait for Module to stop?"=FALSE} ("Stop Argument"), Variant=w288) -> (data=w285:T22, error out=w293:errorcluster)
            n119 = call <vilib>:"Clear Errors.vi"("error in (no error)"=w293, "specific error code to clear (0: all)"=w287) -> ("error out"=w295:errorcluster)  [unwired: 4 in, 1 out]
            n120 = control-ref of="This VI"() -> (w284:refnum<vi>)
            n121 = call-dynamic "Delacor_lib_QMH_Release Message Queue.vi"("error in"=w295, "Message Queue"=w291) -> ("error out"=w294:errorcluster)  [unwired: 9 in]
            n122 = call "Handle Exit.vi"("Stop Argument"=w285, "Admin in"=w283, "VI reference"=w284) -> ("error out"=w292:errorcluster)  [unwired: 7 in, 1 out]
            n123 = Merge Errors(w294, w292) -> (w282:errorcluster)
            n124 = call "Stop Module.vi"("error in"=w282) -> ()  [unwired: 10 in, 1 out]
            n125 = call "Stop Module.vi"("error in"=w282) -> ()  [unwired: 10 in, 1 out]
            n126 = call "Stop Module.vi"("error in"=w282) -> ()  [unwired: 10 in, 1 out]
            n127 = call "Stop Module.vi"("error in"=w282) -> ()  [unwired: 10 in, 1 out]
            n128 = call "Error Reported.vi"("Error"=w282) -> ()  [unwired: 10 in, 1 out]
          }
          frame Default {
            # "'Default' case only runs if there is a message that isn't defined in any of the other cases.  Output a programming error."
            n129 = call "Module Name--constant.vi"() -> ("Module Name"=w301:string)  [unwired: 11 in]
            n130 = Format Into String(format string="The invalid message string \"%s\" was received in the Message Handling Loop for module \"%s\".", w302, w301) -> (resulting string=w297:string)  [unwired: 2 in, 1 out]
            n131 = call <vilib>:"Error Cluster From Error Code.vi"("show call chain? (False)"=TRUE, "error message (\"\")"=w297, "error code (0)"=1) -> ("error out"=w304:errorcluster)  [unwired: 6 in]
            n132 = Merge Errors(w305, w304) -> (w306:errorcluster)
          }
        }
        n133 = call-dynamic "Delacor_lib_QMH_Error Handler - Message Handling Loop.vi"("error in"=w153, "Message Queue in"=w152) -> ("dup error in"=w154:errorcluster)  [unwired: 8 in, 1 out]
      }
      n134 = while "DQMH_HELPER_LOOP" {
        shift-right: [w56] -> _
        shift-left: 1000 -> [w55]
        shift-right: [w53] -> w35
        shift-left: w34 -> [w54]
        tunnel: w38 -> [w50]
        shift-right: [w47] -> _
        shift-left: w32 -> [w48]
        shift-right: [w46] -> _
        shift-left: _ -> [w45]
        stop <- w52 stop-if-true
        w49 = "Hardware Monitoring"  # DQMH_HELPER_LOOP_NAME
        # "Hardware Monitoring"
        n135 = event "DQMH_HELPER_EVENT_STRUCTURE" shown="[0] Timeout" {
          selector: w54 -> [_ _ _]
          dyn-events: [_ _ _] -> w53
          timeout: w55 -> [_ _ _]
          tunnel: w55 -> [w61 w82 w86]
          tunnel: [w61 w82 w86] -> w56
          tunnel: [_ _ TRUE] -> w52
          tunnel: [_ _ errorcluster {"status"=FALSE, "code"=0, "source"=""} ("error constant")] -> w51
          tunnel: w50 -> [_ _ _]
          tunnel: w48 -> [w60 _ w83]
          tunnel: [w59 _ _] -> w47
          tunnel: [w57 w81 _] -> w46
          tunnel: w45 -> [w58 _ _]
          event Timeout {
            n136 = event-data() -> ()  [unwired: 1 in, 1 out]
            n137 = disable-structure shown="Enabled" {
              disable-tunnel: w60 -> [w79 w80]
              disable-tunnel: [w75 w80] -> w59
              disable-tunnel: w58 -> [w70 _]
              disable-tunnel: [w70 _] -> w57
              frame Enabled {
                w69 = 100.0 ("y")
                n138 = property class="System Session"(reference=w79) -> (reference out=w75:refnum<k21>, "FreePhysMem"=w77:dbl, "TotalPhysMem"=w78:dbl, "FreeDisk"=w73:dbl, "TotalDisk"=w72:dbl, "SystemResource"=w74:refnum<k20>)  [unwired: 1 in, 1 out]
                n139 = property class="System Hardware"(reference=w74) -> ("CpuLoadTotal"=w64:u32[])  [unwired: 1 in, 2 out]
                n140 = Divide(x=w73, y=w72) -> (x/y=w71:dbl)
                n141 = Divide(x=w77, y=w78) -> (x/y=w76:dbl)
                n142 = Multiply(x=w76, y=w69) -> (x*y=w66:dbl)
                n143 = Multiply(x=w71, y=w69) -> (x*y=w65:dbl)
                n144 = Index Array(array=w64) -> (element #1=w63:u32, element #2=w62:u32)  [unwired: 2 in]
                n145 = Bundle By Name(cluster=T20 {"Memory RAM Free (%)"=0.0, "Memory ROM Free (%)"=0.0, "CPU 1 (%)"=0, "CPU 2 (%)"=0} ("element"), "Memory RAM Free (%)"=w66, "Memory ROM Free (%)"=w65, "CPU 1 (%)"=w63, "CPU 2 (%)"=w62) -> (w67:T20)
                n146 = RT FIFO Write(0:w70, 1:w67) -> ()  [unwired: 3 in, 4 out]
              }
              frame Disabled {
              }
            }
          }
          event User Event {
            n147 = event-data() -> ("RT FIFO"=w81:refnum<k33>)  [unwired: 1 in]
          }
          event User Event {
            n148 = event-data() -> ()  [unwired: 1 in, 1 out]
            n149 = call-poly <vilib>:"Close.vi"("Session in"=w83) -> ()  [unwired: 10 in, 1 out]
          }
        }
        n150 = call-dynamic "Delacor_lib_QMH_Error Handler - Helper Loop.vi"("Error Debug"=w49, "error in"=w51, "Message Queue in"=w50) -> ()  [unwired: 7 in, 2 out]
      }
      n151 = Unregister For Events(event registration refnum=w35) -> ()  [unwired: 1 in, 1 out]
    }
    frame Error {
      # "Synchronize Caller Events.vi will inform Start Module.vi that the module has launched and will let the code calling Start Module.vi register for broadcasts and would permit the caller receive the broadcast that an error occurred at launch time."
      n152 = call-dynamic "Delacor_lib_QMH_Release Message Queue.vi"("error in"=w314, "Message Queue"=w307) -> ("error out"=w313:errorcluster)  [unwired: 9 in]
      n153 = call "Synchronize Caller Events.vi"("Singleton Module Admin in"=w308) -> ("error out"=w315:errorcluster)  [unwired: 9 in, 1 out]
      n154 = call "Module Name--constant.vi"() -> ("Module Name"=w311:string)  [unwired: 11 in]
      n155 = Format Into String(format string="An error occurred during initialization. %s is no longer running.", w311) -> (resulting string=w309:string)  [unwired: 2 in, 1 out]
      n156 = Merge Errors(w313, w315) -> (w316:errorcluster)
      n157 = call "Error Reported.vi"("Additional Information"=w309, "Error"=w316) -> ()  [unwired: 9 in, 1 out]
    }
  }
  n158 = Merge Errors(w28, w31) -> (w27:errorcluster)
  n159 = call "Close Module.vi"("error in"=w27, "Module Admin in"=w23) -> ("error out"=w29:errorcluster, "External Launch"=w17:bool, "Module Admin out"=w18:refnum<class "Delacor_lib_QMH_Module Admin.lvclass">)  [unwired: 7 in]
  n160 = Unregister For Events(event registration refnum=w22, error in=w29) -> (error out=w26:errorcluster)
  "error out" <- w26
  n161 = case "External Launch?" shown="True" w17 {
    tunnel: w26 -> [_ w317]
    frame False {
    }
    frame True {
      n162 = case shown="No Error" w317 {
        frame No Error {
          n163 = invoke on="Invoke Node" class="VI" method="FP.Close"() -> ()  [unwired: 3 in, 3 out]
        }
        frame Error {
          n164 = disable-structure shown="Default" {
            frame condition #0 (active) {
              n165 = invoke class="VI" method="FP.Open"("Activate"=TRUE ("Activate?")) -> ()  [unwired: 4 in, 5 out]
            }
            frame condition #1 {
              # "Don't show panel on error if running inside a built EXE."
            }
          }
        }
      }
    }
  }
  n166 = local write "Module Admin"(w18) -> ()
